vi "MCCMSG Find Next Multi Clamp.vi"(0 "hMCCmsg":i32, 1 "puModel":u32, 2 "pszSerialNum":string, 3 "uBufSize":u32, 4 "puCOMPortID":u32, 5 "puDeviceID":u32, 6 "puChannelID":u32, 7 "error in (no error)":errorcluster, 8 "pnError":i32) -> (18 "pnError out":i32, 20 "function return":i32, 21 "puModel out":u32, 22 "pszSerialNum out":string, 24 "puCOMPortID out":u32, 25 "puDeviceID out":u32, 26 "puChannelID out":u32, 27 "error out":errorcluster)   [LabVIEW 2012, in "MultiClamp 700B Controls.lvlib" / "AxMultiClampMsg.lvlib"]
doc: "AXMCCMSG BOOL WINAPI MCCMSG_FindNextMultiClamp(HMCCMSG hMCCmsg, UINT *puModel, char *pszSerialNum, UINT uBufSize, UINT *puCOMPortID, UINT *puDeviceID, UINT *puChannelID, int *pnError);"
uses:
  AxMultiClampMsg.lvlib
  AxMultiClampMsg.dll
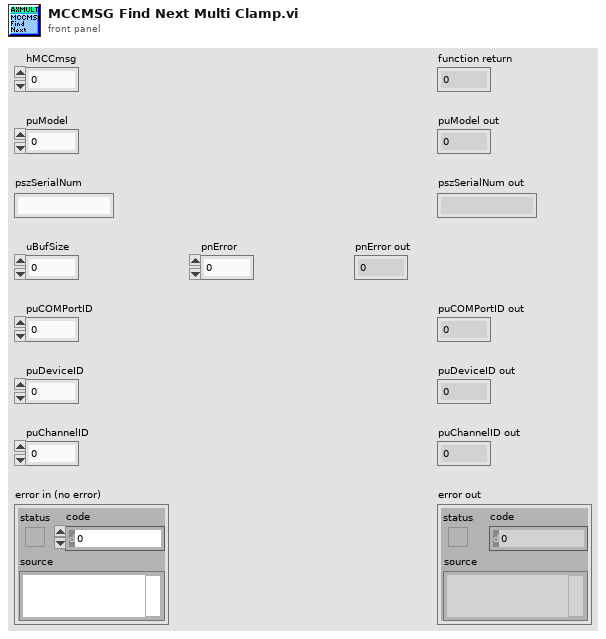
[diagram p1: front panel]
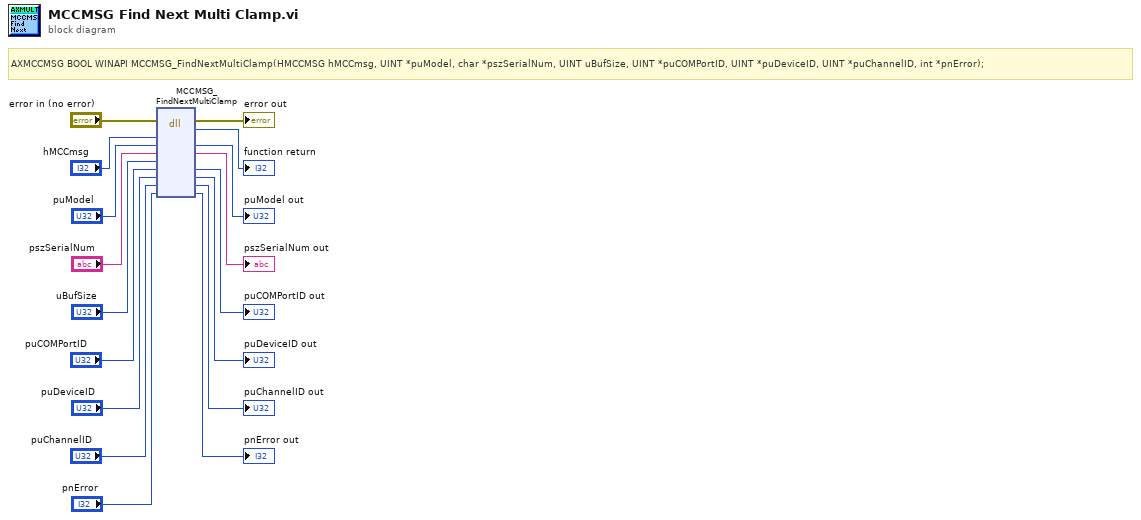
[diagram p0: block diagram]
diagram:
  # "AXMCCMSG BOOL WINAPI MCCMSG_FindNextMultiClamp(HMCCMSG hMCCmsg, UINT *puModel, char *pszSerialNum, UINT uBufSize, UINT *puCOMPortID, UINT *puDeviceID, UINT *puChannelID, int *pnError);"
  n1 = dll-call lib="C:/Users/LAA12/Desktop/Rita/Multiclamp 700B VIs/AxMultiClampMsg/AxMultiClampMsg.*" fn="MCCMSG_FindNextMultiClamp"(error in="error in (no error)", "hMCCmsg"="hMCCmsg", "puModel"="puModel", "pszSerialNum"="pszSerialNum", "uBufSize"="uBufSize", "puCOMPortID"="puCOMPortID", "puDeviceID"="puDeviceID", "puChannelID"="puChannelID", "pnError"="pnError") -> (error out=→"error out":errorcluster, →"function return":i32, "puModel"=→"puModel out":u32, "pszSerialNum"=→"pszSerialNum out":string, "puCOMPortID"=→"puCOMPortID out":u32, "puDeviceID"=→"puDeviceID out":u32, "puChannelID"=→"puChannelID out":u32, "pnError"=→"pnError out":i32)  [unwired: 4 in, 1 out]
